vi "DHE_Lib_stop_integrate.vi"(11 "error in (no error)":errorcluster) -> (6 "actual integ":i32, 15 "error out":errorcluster)   [LabVIEW 2016]
doc: "This VI opens (Flag=1) or closes (Flag=0) the instrument shutter."
uses:
  c/lib/libgendhe.so
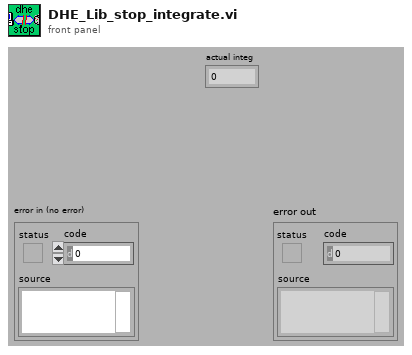
[diagram p1: front panel]
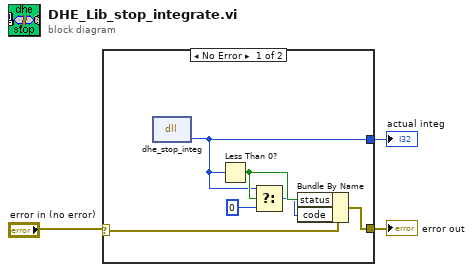
[diagram p0: block diagram]
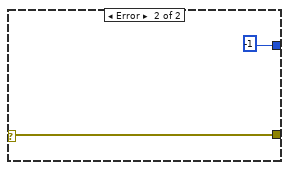
[diagram p2: hidden frame]
diagram:
  n1 = case shown="No Error" "error in (no error)" {
    selector: "error in (no error)" -> [w9 w11]
    tunnel: [w8 w11] -> w3
    tunnel: [w6 -1] -> w1
    frame No Error {
      n2 = dll-call lib="uyq0/bonati/panview_lv14/PAN/Modules/DHE/private/c/lib/libgendhe.so" fn="dhe_stop_integ"() -> ("return type"=w6:i32)  [unwired: 3 in, 2 out]
      n3 = Less Than 0?(x=w6) -> (x < 0?=w7:bool)
      n4 = Select(t=w6, s=w7, f=0) -> (s? t:f=w5:i32)
      n5 = Bundle By Name(cluster=w9, "status"=w7, "code"=w5) -> (w8:errorcluster)
    }
    frame Error {
    }
  }
  "error out" <- w3
  "actual integ" <- w1
